vi "Actor Core.vi"(8 "error in":errorcluster, 11 "RDS Root Actor in":refnum<class "RDS Root Actor.lvclass">) -> (0 "error out":errorcluster, 3 "Actor out":refnum<class "Actor.lvclass">)   [LabVIEW 2015, in "RDS Root Actor.lvlib" / "RDS Root Actor.lvclass"]
doc: "(<B>Filename</B>: Actor Framework.lvlib:Actor.lvclass:Actor Core.vi)\n\nReceives messages to the actor, reacts to them, and initiates any error handling that may shut the actor down.\n\nDescendant classes may override this VI to append parallel tasks for the actor to complete while it handles messages. Overrides use the Call Parent Method node."
uses:
  RDS Root Actor.lvclass
  <vilib>/ActorFramework/Actor/Actor.lvclass
  RDS Router Actor/RDS Router Actor/RDS Router Actor.lvclass
  RDS Root Actor.lvclass/RDS Root Actor.ctl
  RDS Parent Actor/RDS Parent Actor Messages/RDS Post Launch Init Msg/RDS Post Launch Init Msg.lvclass
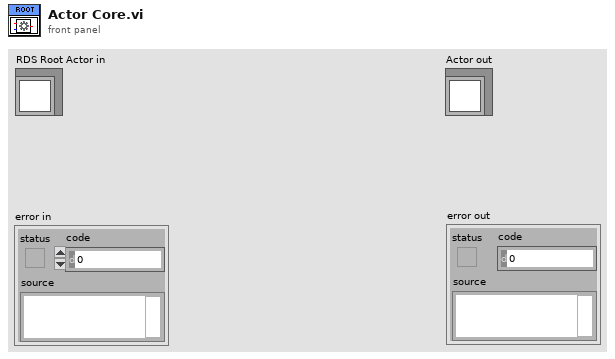
[diagram p1: front panel]
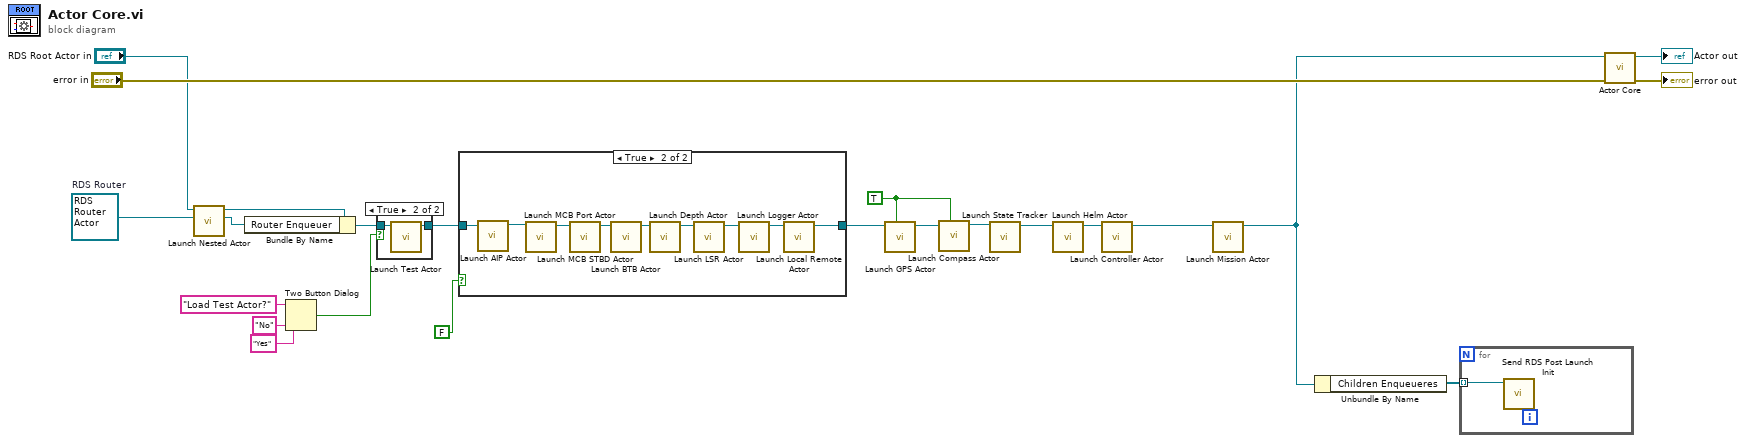
[diagram p0: block diagram]
diagram:
  w4 = TRUE ("Sim?")
  w19 = refnum<class "RDS Router Actor.lvclass"> refnum  # RDS Router
  n1 = call <vilib>:"Launch Nested Actor.vi"("Nested Actor"=w19, "Caller Actor in"="RDS Root Actor in") -> ("Nested Actor's Enqueuer"=w17:refnum<class "Message Enqueuer.lvclass">, "Caller Actor out"=w18:refnum<class "RDS Root Actor.lvclass">)  [unwired: 7 in, 1 out]
  n2 = Bundle By Name(cluster=w18, "Router Enqueuer"=w17) -> (w20:refnum<class "RDS Root Actor.lvclass">)
  n3 = Two Button Dialog(message="Load Test Actor?", 1:"No" ("F button name (\"Cancel\")"), 2:"Yes" ("T button name (\"OK\")")) -> (T button?=w10:bool)
  n4 = case shown="True" w10 {
    tunnel: w20 -> [w24 w26]
    tunnel: [w24 w25] -> w14
    frame False {
    }
    frame True {
      n5 = call "Launch Test Actor.vi"("RDS Root Actor in"=w26) -> ("RDS Root Actor out"=w25:refnum<class "RDS Root Actor.lvclass">)  [unwired: 10 in]
    }
  }
  n6 = case shown="True" FALSE {
    tunnel: w14 -> [w27 w32]
    tunnel: [w27 w28] -> w7
    frame False {
    }
    frame True {
      n7 = call "Launch AIP Actor.vi"("RDS Root Actor in"=w32) -> ("RDS Root Actor out"=w31:refnum<class "RDS Root Actor.lvclass">)  [unwired: 10 in]
      n8 = call "Launch MCB Port Actor.vi"("RDS Root Actor in"=w31) -> ("RDS Root Actor out"=w36:refnum<class "RDS Root Actor.lvclass">)  [unwired: 10 in]
      n9 = call "Launch MCB STBD Actor.vi"("RDS Root Actor in"=w36) -> ("RDS Root Actor out"=w35:refnum<class "RDS Root Actor.lvclass">)  [unwired: 10 in]
      n10 = call "Launch BTB Actor.vi"("RDS Root Actor in"=w35) -> ("RDS Root Actor out"=w34:refnum<class "RDS Root Actor.lvclass">)  [unwired: 10 in]
      n11 = call "Launch Depth Actor.vi"("RDS Root Actor in"=w34) -> ("RDS Root Actor out"=w33:refnum<class "RDS Root Actor.lvclass">)  [unwired: 10 in]
      n12 = call "Launch LSR Actor.vi"("RDS Root Actor in"=w33) -> ("RDS Root Actor out"=w30:refnum<class "RDS Root Actor.lvclass">)  [unwired: 10 in]
      n13 = call "Launch Logger Actor.vi"("RDS Root Actor in"=w30) -> ("RDS Root Actor out"=w29:refnum<class "RDS Root Actor.lvclass">)  [unwired: 10 in]
      n14 = call "Launch Local Remote Actor.vi"("RDS Root Actor in"=w29) -> ("RDS Root Actor out"=w28:refnum<class "RDS Root Actor.lvclass">)  [unwired: 10 in]
    }
  }
  n15 = call "Launch GPS Actor.vi"("Sim?"=w4, "RDS Root Actor in"=w7) -> ("RDS Root Actor out"=w6:refnum<class "RDS Root Actor.lvclass">)  [unwired: 9 in]
  n16 = call "Launch Compass Actor.vi"("Sim?"=w4, "RDS Root Actor in"=w6) -> ("RDS Root Actor out"=w5:refnum<class "RDS Root Actor.lvclass">)  [unwired: 9 in]
  n17 = call "Launch State Tracker.vi"("RDS Root Actor in"=w5) -> ("RDS Root Actor out"=w2:refnum<class "RDS Root Actor.lvclass">)  [unwired: 10 in]
  n18 = call "Launch Helm Actor.vi"("RDS Root Actor in"=w2) -> ("RDS Root Actor out"=w12:refnum<class "RDS Root Actor.lvclass">)  [unwired: 10 in]
  n19 = call "Launch Controller Actor.vi"("RDS Root Actor in"=w12) -> ("RDS Root Actor out"=w1:refnum<class "RDS Root Actor.lvclass">)  [unwired: 10 in]
  n20 = call "Launch Mission Actor.vi"("RDS Root Actor in"=w1) -> ("RDS Root Actor out"=w3:refnum<class "RDS Root Actor.lvclass">)  [unwired: 10 in]
  n21 = Unbundle By Name(w3) -> ("Children Enqueueres"=w16:refnum<class "Message Enqueuer.lvclass">[])
  n22 = for {
    tunnel: w16 -> [w37] mode=indexing
    n23 = call "Send RDS Post Launch Init.vi"("Message Enqueuer in"=w37) -> ()  [unwired: 9 in, 2 out]
  }
  n24 = call-parent "Actor Core.vi"("error in"="error in", "Actor in"=w3) -> ("error out"=→"error out":errorcluster, "Actor out"=→"Actor out":refnum<class "Actor.lvclass">)  [unwired: 8 in]
